vi "Write Transport Options.vi"(8 "error in (no error)":errorcluster, 10 "Transport Options":T1, 11 "WAMP Client in":refnum<class "WAMP Client.lvclass">) -> (0 "error out":errorcluster, 3 "WAMP Client out":refnum<class "WAMP Client.lvclass">)   [LabVIEW 2020, in "wamplv.lvlib" / "WAMP Client.lvclass"]
uses:
  WAMP Client.lvclass
  API/TypeDefs/Transport Options.ctl
  Private/Comm Handlers/Websocket Handler/Options.ctl
  Private/Comm Handlers/Websocket Handler/Headers.ctl
  WAMP Client.lvclass/WAMP Client.ctl
  Private/Comm Handlers/Websocket Handler/Websocket Handler.lvclass
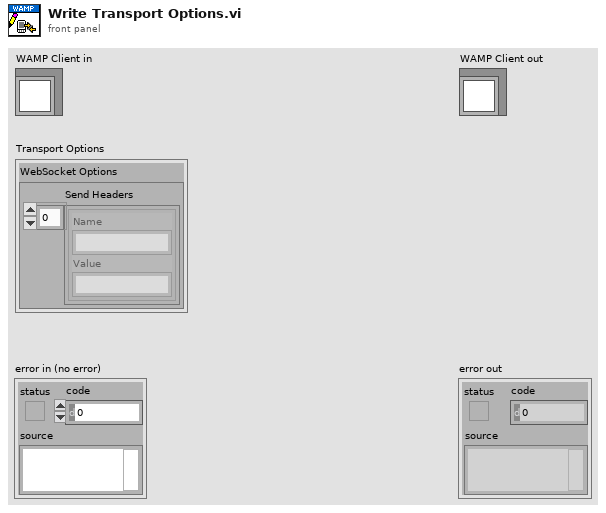
[diagram p1: front panel]
types:
  T1 = typedef "wamplv.lvlib/WAMP Client.lvclass/Transport Options.ctl" = cluster{"WebSocket Options":T2}
  T2 = typedef "wamplv.lvlib/Websocket Handler.lvclass/Options.ctl" = cluster{"Send Headers":T3[]}
  T3 = typedef "wamplv.lvlib/Websocket Handler.lvclass/Headers.ctl" = cluster{"Name":string, "Value":string}
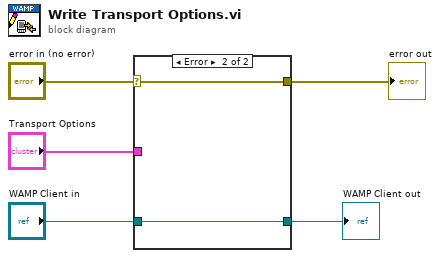
[diagram p0: block diagram]
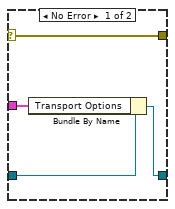
[diagram p2: hidden frame]
diagram:
  n1 = case shown="Error" "error in (no error)" {
    selector: "error in (no error)" -> [w6 w10]
    tunnel: [w6 w10] -> w4
    tunnel: [w7 w11] -> w2
    tunnel: "WAMP Client in" -> [w9 w11]
    tunnel: "Transport Options" -> [w8 _]
    frame No Error {
      n2 = Bundle By Name(cluster=w9, "Transport Options"=w8) -> (w7:refnum<class "WAMP Client.lvclass">)
    }
    frame Error {
    }
  }
  "error out" <- w4
  "WAMP Client out" <- w2
